vi "Test_Benchmarking_LogEventCall_AvgCallTimeSub10uS.vi"(8 "error in (no error)":errorcluster, 11 "Benchmarking in":refnum<class "Benchmarking.lvclass">) -> (0 "error out":errorcluster, 3 "Benchmarking out":refnum<class "Benchmarking.lvclass">)   [LabVIEW 2017, in "Benchmarking.lvclass"]
uses:
  Benchmarking.lvclass
  Source/Composed Log/LoggerReference/LoggerReference.lvclass/LoggerReference.ctl
  Source/Composed Log/Types/Log Level.ctl
  9d967267-f109-4650-a18c-21849a313d7c.vi
  <vilib>/Analysis/baseanly.llb/Mean (DBL).vi
  9d967267-f109-4650-a18c-21849a313d7c.vi/fefadb42-e23f-461b-ac24-2aaf4d3ea4d3.vi
  Source/Composed Log/LoggerReference/Return Aggregate Queues.vi
  Source/Composed Log/LoggerReference/Add Aggregate Log.vi
  9d967267-f109-4650-a18c-21849a313d7c.vi/fefadb42-e23f-461b-ac24-2aaf4d3ea4d3.vi/bb3a4a6e-475e-47a3-8423-93e32af95be7.vi
  Source/Composed Log/LoggerReference/Log.vi
  Source/Composed Log/LoggerReference/Send Add Sink.vi
  Source/Composed Log/LoggerReference/Remove Stale Logs.vi
  Source/LVQueue Sink/LVQueue Sink.lvclass
  C:/CS/Internal/LabVIEW/Logger/Source/Composed Log/Log Sink/Log Sink.lvclass
  Source/Composed Log/Application Logger/Launch Worker Loop.vi
  Source/Composed Log/LoggerReference/Initialize Logger Instance.vi
  Source/Composed Log/Singleton Event Log/Logger Queue FGV.vi
  Source/Composed Log/IErrorFormat/IErrorFormat.lvclass
  Source/Composed Log/LoggerReference/LoggerReference.lvclass
  Source/Composed Log/Log Sink/Log Sink.lvclass
  Source/Composed Log/Singleton Event Log/Singleton Event Log.lvlib
  <vilib>/Analysis/NI_AALBase.lvlib
  <vilib>/addons/_JKI Toolkits/VI Tester/TestCase.llb/TestCase.lvclass
  Source/Composed Log/Composed Log.lvlib
  C:/Program Files (x86)/National Instruments/LabVIEW 2017/vi.lib/addons/_JKI Toolkits/VI Tester/TestCase.llb/TestCase.lvclass
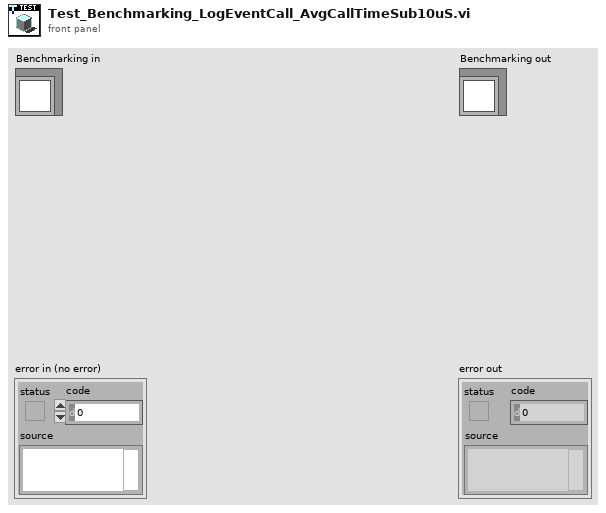
[diagram p1: front panel]
types:
  T1 = typedef "Composed Log.lvlib/Log Level.ctl" = enum16{"Debug", "Info", "Warning", "Error", "Critical"}
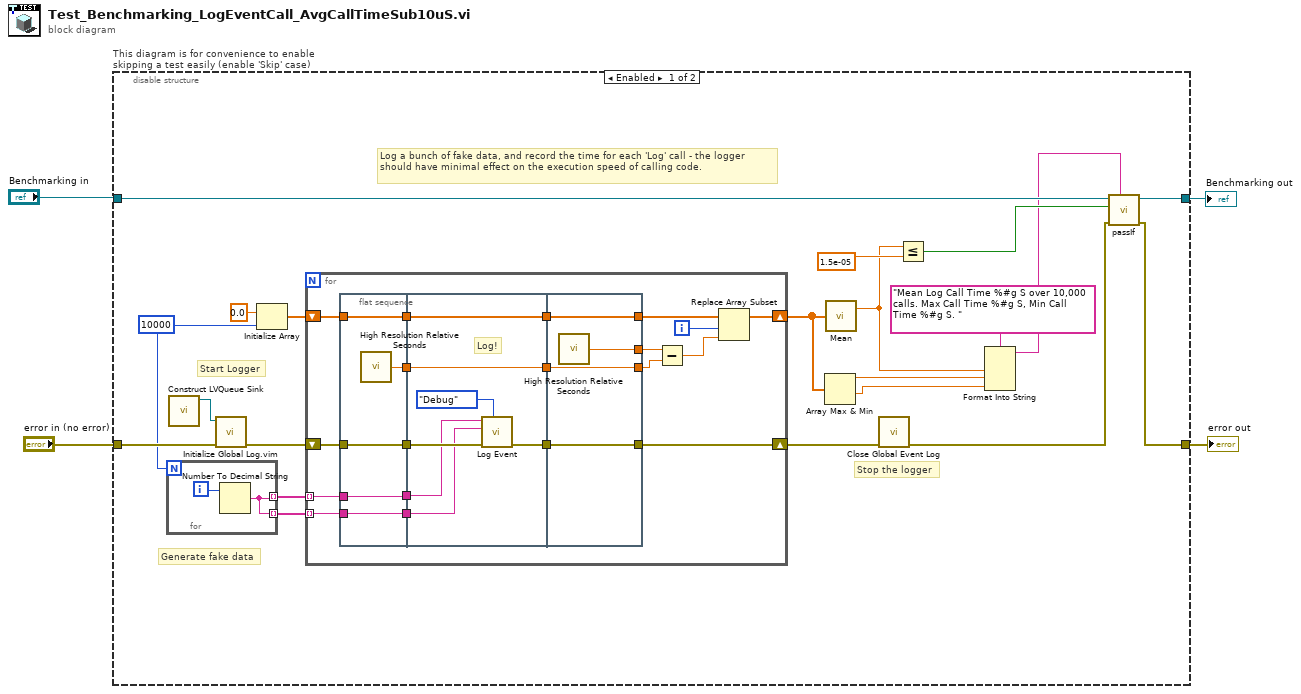
[diagram p0: block diagram]
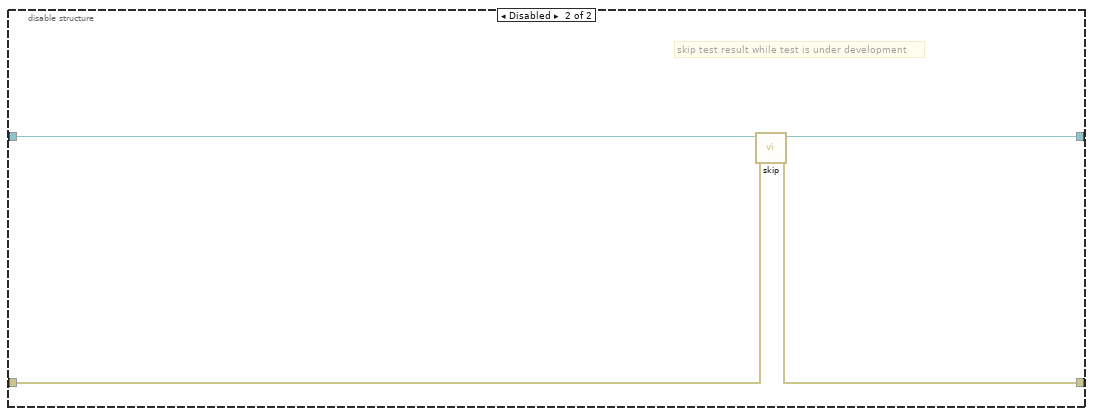
[diagram p2: hidden frame]
diagram:
  n1 = disable-structure "This diagram is for convenience to enable skipping a test easily (enable 'Skip' case)" shown="Enabled" {
    disable-tunnel: "Benchmarking in" -> [w15 w66]
    disable-tunnel: [w14 w64] -> w4
    disable-tunnel: [w16 w65] -> w3
    disable-tunnel: "error in (no error)" -> [w25 w63]
    frame Enabled {
      w21 = 10000
      # "Stop the logger"
      # "Generate fake data"
      # "Start Logger"
      # "Log a bunch of fake data, and record the time for each 'Log' call - the logger should have minimal effect on the execution speed of calling code."
      n2 = for {
        N: w21 -> [_]
        tunnel: [w61] -> w24 mode=indexing
        tunnel: [w61] -> w13 mode=indexing
        i -> [w62]
        n3 = Number To Decimal String(number=w62) -> (decimal integer string=w61:string)  [unwired: 1 in]
      }
      n4 = call "Construct LVQueue Sink.vi"() -> ("LVQueue Sink out"=w5:refnum<class "LVQueue Sink.lvclass">)  [unwired: 10 in, 1 out]
      n5 = call "Initialize Global Log.vim"("error in (no error)"=w25, "Log Sink(s)"=w5) -> ("error out"=w23:errorcluster)  [unwired: 8 in, 1 out]
      n6 = Initialize Array(0.0 ("element"), w21) -> (w19:dbl[])
      n7 = for {
        tunnel: w24 -> [w39] mode=indexing
        shift-right: [w37] -> w22
        shift-left: w23 -> [w38]
        shift-right: [w28] -> w18
        shift-left: w19 -> [w34]
        tunnel: w13 -> [w27] mode=indexing
        i -> [w30]
        n8 = flat-sequence {
          tunnel: w38 -> [w48]
          tunnel: w39 -> [w49]
          tunnel: [w49] -> w44
          tunnel: [w48] -> w43
          tunnel: [w47] -> w42
          tunnel: w34 -> [w46]
          tunnel: [w46] -> w32
          tunnel: w27 -> [w45]
          tunnel: [w45] -> w26
          tunnel: w44 -> [w53]
          tunnel: w43 -> [w54]
          tunnel: w42 -> [w56]
          tunnel: [w51] -> w41
          tunnel: [w56] -> w40
          tunnel: [w55] -> w33
          tunnel: w32 -> [w55]
          tunnel: w26 -> [w52]
          tunnel: [w59] -> w36
          tunnel: [w60] -> w37
          tunnel: w41 -> [w60]
          tunnel: w40 -> [w59]
          tunnel: [w58] -> w35
          tunnel: [w57] -> w31
          tunnel: w33 -> [w57]
          frame #0 {
            n9 = call <vilib>:"High Resolution Relative Seconds.vi"() -> ("relative seconds"=w47:dbl)
          }
          frame #1 {
            # "Log!"
            n10 = call "Log Event.vi"("Event Level"=Log_Level."Debug", "error in (no error)"=w54, "Data To Log"=w52, "SourceID"=w53) -> ("error out"=w51:errorcluster)  [unwired: 7 in]
          }
          frame #2 {
            n11 = call <vilib>:"High Resolution Relative Seconds.vi"() -> ("relative seconds"=w58:dbl)
          }
        }
        n12 = Subtract(x=w35, y=w36) -> (x-y=w29:dbl)
        n13 = Replace Array Subset(array=w31, new element=w29, index=w30) -> (w28:dbl[])
      }
      n14 = Array Max & Min(array=w18) -> (max value=w8:dbl, min value=w7:dbl)  [unwired: 2 out]
      n15 = call-poly <vilib>:"Mean.vi"("X"=w18) -> ("mean"=w9:dbl)  [unwired: 1 out]
      n16 = call "Close Global Event Log.vi"("error in (no error)"=w22) -> ("error out"=w17:errorcluster)  [unwired: 10 in]
      n17 = Less Or Equal?(x=w9, y=1.5e-05) -> (x <= y?=w11:bool)
      n18 = Format Into String(format string="Mean Log Call Time %#g S over 10,000 calls. Max Call Time %#g S, Min Call Time %#g S. ", w9, w8, w7) -> (resulting string=w6:string)  [unwired: 2 in, 1 out]
      n19 = call-dynamic "passIf.vi"("custom report message (\"\")"=w6, "error in (no error)"=w17, "pass"=w11, "TestCase in"=w15) -> ("error out"=w16:errorcluster, "TestCase out"=w14:refnum<class "Benchmarking.lvclass">)  [unwired: 6 in]
    }
    frame Disabled {
      # "skip test result while test is under development"
      n20 = call <vilib>:"skip.vi"("error in (no error)"=w63, "TestCase in"=w66) -> ("error out"=w65:errorcluster, "TestCase out"=w64:refnum<class "Benchmarking.lvclass">)  [unwired: 8 in]
    }
  }
  "error out" <- w3
  "Benchmarking out" <- w4
